vi "Slider Simulation Details (SubVI).vi"(7 "Number of Steps":u32) -> (0 "Time Between Steps (ms)":dbl, 3 "Step Size (mm)":dbl)   [LabVIEW 2012]
uses:
  Stage Global.vi
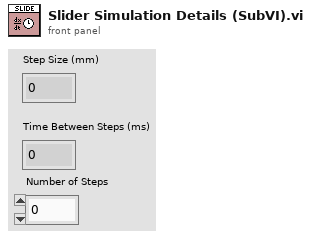
[diagram p1: front panel]
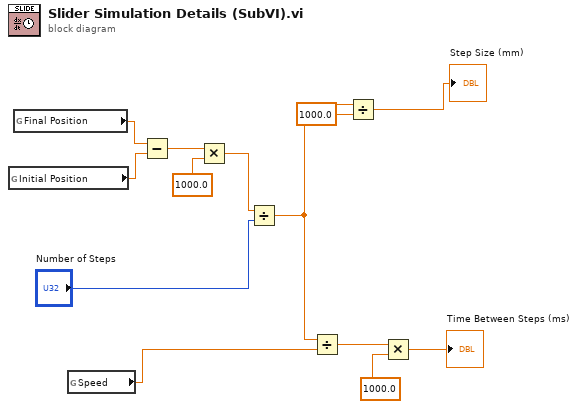
[diagram p0: block diagram]
diagram:
  n1 = global read "Stage Global.vi" "Initial Position"() -> (w6:dbl)
  n2 = global read "Stage Global.vi" "Final Position"() -> (w7:dbl)
  n3 = global read "Stage Global.vi" "Speed"() -> (w9:dbl)
  n4 = Subtract(x=w7, y=w6) -> (x-y=w5:dbl)
  n5 = Multiply(x=w5, y=1000.0 ("x")) -> (x*y=w4:dbl)
  n6 = Divide(x=w4, y="Number of Steps") -> (x/y=w3:dbl)
  n7 = Divide(x=w3, y=w9) -> (x/y=w12:dbl)
  n8 = Divide(x=w3, y=1000.0) -> (x/y=→"Step Size (mm)":dbl)
  n9 = Multiply(x=w12, y=1000.0) -> (x*y=→"Time Between Steps (ms)":dbl)
